vi "OCR Control.vi"() -> ()   [LabVIEW 2014]
uses:
  Resources/Global.vi
  <vilib>/vision/NI_Vision_Development_Module.lvlib
panel:
  out "Command string":string
  out "State":string
  out "Land/TakeOff":bool
  out "Get Video Stream Error":errorcluster
  out "OCR":T1(plugin-control)
  out "Number of Lines":i32
  out "Read String":string
  in  "error in (no error)":errorcluster
  # "Do NOT run this VI. Instead run \"AR.Drone MAIN.vi\" and select the name of this VI in the dop-down menu at the Steup tab"
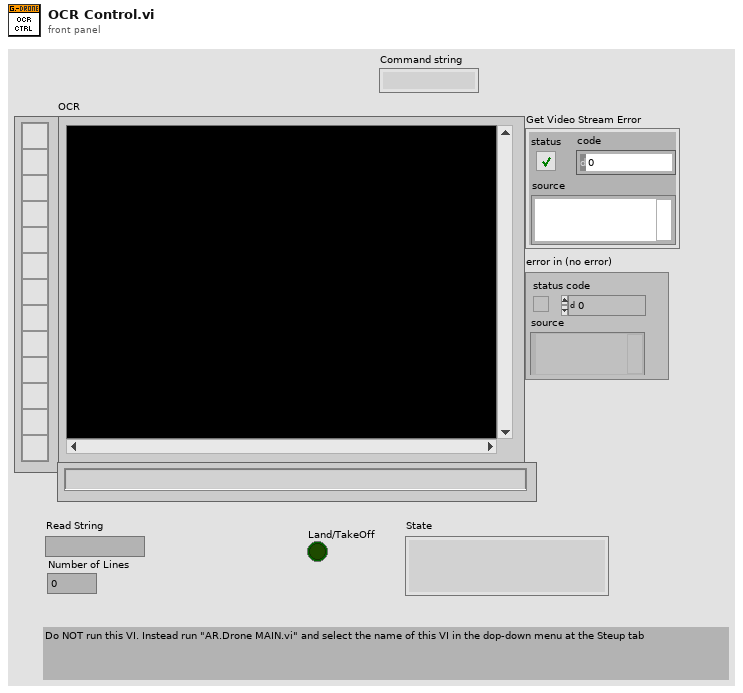
[diagram p1: front panel]
types:
  T1 = typedef "IMAQ Image.ctl" = refnum<image>
  T2 = typedef "Image Type" = u32
  T3 = typedef "IMAQ OCR Session.ctl" = refnum<k1>
  T4 = cluster{"Desired Font (Application)":enum16{"User-specified Font", "Application Font", "System Font", "Dialog Font"}, "[User-specified Font]":cluster{"Font Name":string, "Size":i16, "Strikeout?":bool, "Italic?":bool, "Underline?":bool, "Outline?":bool, "Shadow?":bool, "Bold?":bool, "Rotation Angle":dbl}, "Horizontal Alignment":i16, "Vertical Alignment":i16}
  T5 = cluster{"Global Rectangle":i32[], "Contours":cluster{"ID":enum32{"External", "Internal"}, "Type":u32, "Coordinates":i32[]}[]}
  T6 = typedef "Control cluster.ctl" = cluster{"Roll":sgl, "Pitch":sgl, "Vertical Speed":sgl, "Yaw Speed":sgl}
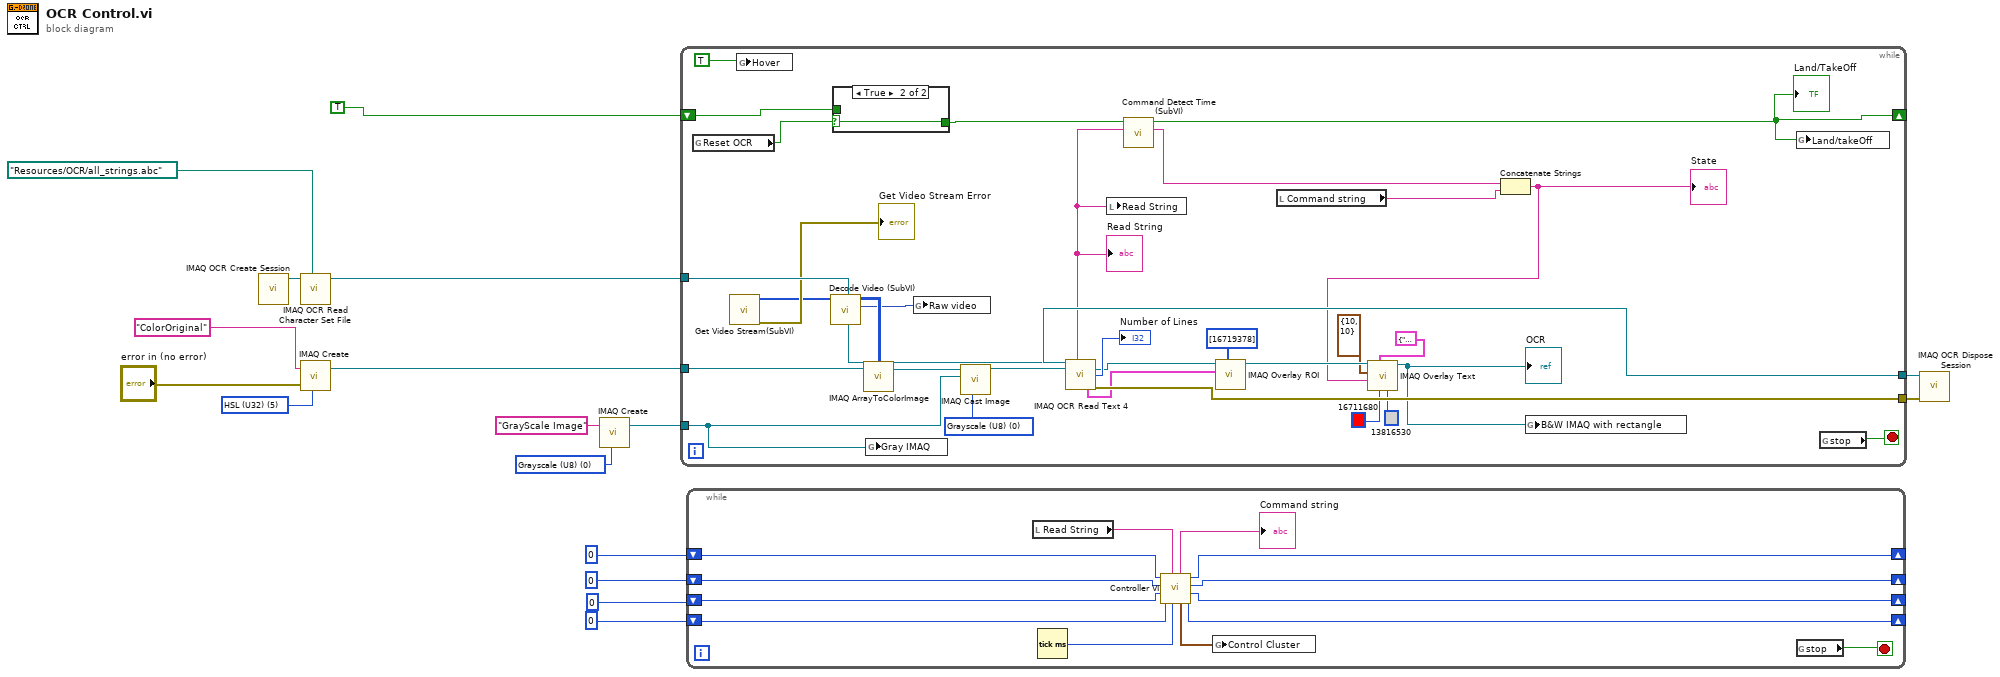
[diagram p0: block diagram]
diagram:
  w3 = T2 0 items=["Grayscale (U8)", "Grayscale (I16)", "Grayscale (SGL)", "Complex (CSG)", "RGB (U32)", "HSL (U32)", "RGB (U64)", "Grayscale (U16)"] ("Image Type")
  w17 = T2 5 items=["Grayscale (U8)", "Grayscale (I16)", "Grayscale (SGL)", "Complex (CSG)", "RGB (U32)", "HSL (U32)", "RGB (U64)", "Grayscale (U16)"] ("Image Type")
  n1 = call "IMAQ OCR Create Session"() -> ("IMAQ OCR Session"=w12:T3)  [unwired: 10 in, 1 out]
  n2 = call "IMAQ OCR Read Character Set File"("File Path"=path "Resources/OCR/all_strings.abc", "IMAQ OCR Session"=w12) -> ("IMAQ OCR Session (dup)"=w11:T3)  [unwired: 7 in, 2 out]
  n3 = call "IMAQ Create"("Image Name"="ColorOriginal", "Image Type"=w17, "error in (no error)"="error in (no error)") -> ("New Image"=w16:T1)  [unwired: 2 in, 1 out]
  n4 = call "IMAQ Create"("Image Name"="GrayScale Image", "Image Type"=w3) -> ("New Image"=w1:T1)  [unwired: 3 in, 1 out]
  n5 = while {
    tunnel: w16 -> [w40]
    tunnel: [w48] -> w14
    tunnel: [w47] -> w13
    tunnel: w11 -> [w46]
    shift-right: [w36] -> _
    shift-left: TRUE -> [w38]
    tunnel: w1 -> [w19]
    stop <- w34 stop-if-true
    w49 = T2 0 items=["Grayscale (U8)", "Grayscale (I16)", "Grayscale (SGL)", "Complex (CSG)", "RGB (U32)", "HSL (U32)", "RGB (U64)", "Grayscale (U16)"] ("Image Type")
    n6 = global read "Global.vi" "Reset OCR"() -> (w18:bool)
    n7 = call "Get Video Stream(SubVI).vi"() -> ("error out"=→"Get Video Stream Error":errorcluster, "ImgData"=w31:u8[])  [unwired: 10 in]
    n8 = global write "Global.vi" "Hover"(TRUE ("Hover")) -> ()
    n9 = call "Decode Video (SubVI).vi"("ImgData"=w31) -> ("new picture"=w29:picture, "Array"=w30:u32[][])  [unwired: 9 in]
    n10 = case shown="True" w18 {
      selector: w18 -> [_ w51]
      tunnel: w38 -> [w50 _]
      tunnel: [w50 w51] -> w37
      frame False {
      }
      frame True {
      }
    }
    n11 = call "IMAQ ArrayToColorImage"("Image Pixels (U32)"=w30, "Image"=w40) -> ("Image Out"=w41:T1)  [unwired: 3 in, 1 out]
    n12 = global write "Global.vi" "Gray IMAQ"(w19) -> ()
    n13 = global write "Global.vi" "Raw video"(w29) -> ()
    n14 = call "IMAQ Cast Image"("Image Type"=w49, "Image Dst"=w19, "Image Src"=w41) -> ("Image Dst Out"=w23:T1)  [unwired: 7 in, 1 out]
    n15 = call "IMAQ OCR Read Text 4"("IMAQ OCR Session"=w46, "Image"=w23) -> ("IMAQ OCR Session (dup)"=w47:T3, "Image (dup)"=w42:T1, "Number of Lines"=→"Number of Lines":i32, "Read String"=w33:string, "ROI Bounding Characters"=w44:T5, "error out"=w48:errorcluster)  [unwired: 7 in, 1 out]
    "Read String" <- w33
    n16 = local write "Read String"(w33) -> ()
    n17 = call "Command Detect Time (SubVI).vi"("Read String"=w33, "Boolean in"=w37) -> ("String"=w32:string, "Boolean out"=w36:bool)  [unwired: 8 in]
    "Land/TakeOff" <- w36
    n18 = call "IMAQ Overlay ROI"("Colors (Green)"=u32[] [16719378], "ROI Descriptor"=w44, "Image"=w42) -> ("Image Out"=w28:T1)  [unwired: 7 in, 1 out]
    n19 = local read "Command string"() -> (w20:string)
    n20 = Concatenate Strings(w32, w20) -> (w26:string)
    "State" <- w26
    n21 = call "IMAQ Overlay Text"("BG Color (Transparent)"=u32 13816530, "Text Color (black)"=u32 16711680, "Font, Size & Style"=T4 {"Desired Font (Application)"=enum."User-specified Font", "[User-specified Font]"={"Font Name"="Calibri", "Size"=30, "Strikeout?"=FALSE, "Italic?"=FALSE, "Underline?"=FALSE, "Outline?"=TRUE, "Shadow?"=TRUE, "Bold?"=TRUE, "Rotation Angle"=0.0}, "Horizontal Alignment"=0, "Vertical Alignment"=1}, "String"=w26, "Origin"=cluster{"X":i32, "Y":i32} {"X"=10, "Y"=10}, "Image"=w28) -> ("Image Out"=w27:T1)  [unwired: 4 in, 1 out]
    "OCR" <- w27
    n22 = global write "Global.vi" "B&W IMAQ with rectangle"(w27) -> ()
    n23 = global write "Global.vi" "Land/takeOff"(w36) -> ()
    n24 = global read "Global.vi" "stop"() -> (w34:bool)
  }
  n25 = while {
    shift-right: [w56] -> _
    shift-left: u32 0 ("millisecond timer value") -> [w52]
    shift-right: [w58] -> _
    shift-left: u32 0 ("millisecond timer value") -> [w54]
    shift-right: [w57] -> _
    shift-left: u32 0 ("millisecond timer value") -> [w53]
    shift-right: [w59] -> _
    shift-left: u32 0 ("millisecond timer value") -> [w55]
    stop <- w64 stop-if-true
    n26 = local read "Read String"() -> (w61:string)
    n27 = Tick Count (ms)() -> (millisecond timer value=w62:u32)
    n28 = call "Controller VI.vi"("Current Time In"=w62, "Read String"=w61, "Down Detect Time In"=w52, "Up Detect Time In"=w53, "Left Detect Time In"=w54, "Right Detect Time In"=w55) -> ("Down Detect Time Out"=w56:u32, "Up Detect Time Out"=w57:u32, "Left Detect Time Out"=w58:u32, "Right detect Time Out"=w59:u32, "Control Cluster"=w63:T6, "Command string"=→"Command string":string)
    n29 = global write "Global.vi" "Control Cluster"(w63) -> ()
    n30 = global read "Global.vi" "stop"() -> (w64:bool)
  }
  n31 = call "IMAQ OCR Dispose Session"("error in (no error)"=w14, "IMAQ OCR Session"=w13) -> ()  [unwired: 9 in, 1 out]
